vi "createModbusSubnetE.vi"(8 "error in (no error)":errorcluster, 11 "Boot in":refnum<class "Boot.lvclass">) -> (0 "error out":errorcluster, 2 "ModbusSubnetE":refnum<class "IModbus.lvclass">, 3 "Boot out":refnum<class "Boot.lvclass">)   [LabVIEW 2016, in "Boot.lvclass"]
uses:
  Boot.lvclass
  Common_RT_Modbus/IModbus/IModbus.lvclass
  Common_RT_Modbus/Modbus/Modbus.lvclass
  D:/Code/ts_M1M3Support/Common_RT_Modbus/IModbus/IModbus.lvclass
  Resources/ModbusSubnetETxDataFIFO/ModbusSubnetETxDataFIFO.lvclass
  D:/Code/ts_M1M3Support/Common_RT_FPGA/IWriteU16FIFO/IWriteU16FIFO.lvclass
  Boot.lvclass/Boot.ctl
  Resources/ModbusSubnetETxDataFIFO/ModbusSubnetETxDataFIFO.lvclass/ModbusSubnetETxDataFIFO.ctl
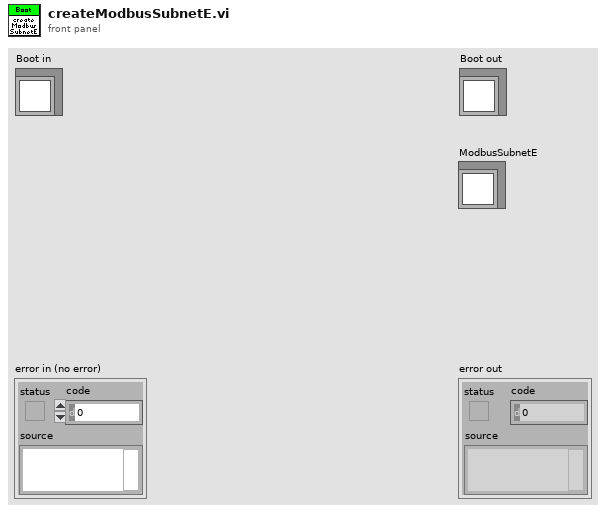
[diagram p1: front panel]
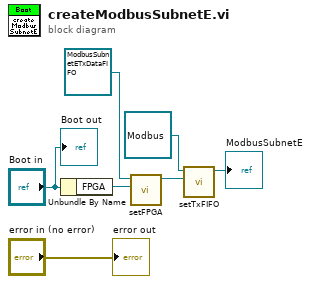
[diagram p0: block diagram]
diagram:
  n1 = Unbundle By Name("Boot in") -> ("FPGA"=w2:refnum<class "FPGA.lvclass">)
  n2 = call "setFPGA.vi"("FPGA"=w2, "ModbusSubnetETxDataFIFO in"=refnum<class "ModbusSubnetETxDataFIFO.lvclass"> refnum ("ModbusSubnetETxDataFIFO.lvclass")) -> ("ModbusSubnetETxDataFIFO out"=w1:refnum<class "ModbusSubnetETxDataFIFO.lvclass">)  [unwired: 9 in]
  n3 = call "setTxFIFO.vi"("WriteU16FIFO"=w1, "Modbus in"=refnum<class "Modbus.lvclass"> refnum ("RTModbus.lvlib:Modbus.lvclass")) -> ("Modbus out"=→"ModbusSubnetE":refnum<class "Modbus.lvclass">)  [unwired: 9 in]
  "error out" <- "error in (no error)"
  "Boot out" <- "Boot in"
